vi "CreateProgram.vi"() -> ()   [LabVIEW 2018]
panel:
  out "error out":errorcluster
  in  "Clear":bool
  in  "Save":bool
  in  "Loop End":bool
  in  "Loop Start":bool
  in  "Incubate":bool
  in  "Change Reagent":bool
  in  "Feed":bool
  in  "Pump":bool
  out "Program Steps":i32(listbox)
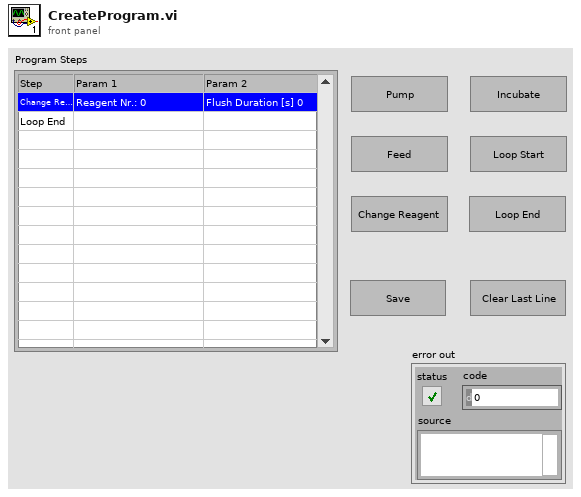
[diagram p1: front panel]
types:
  T1 = enum16{"open", "replace", "create", "open or create", "replace or create", "replace or create with confirmation"}
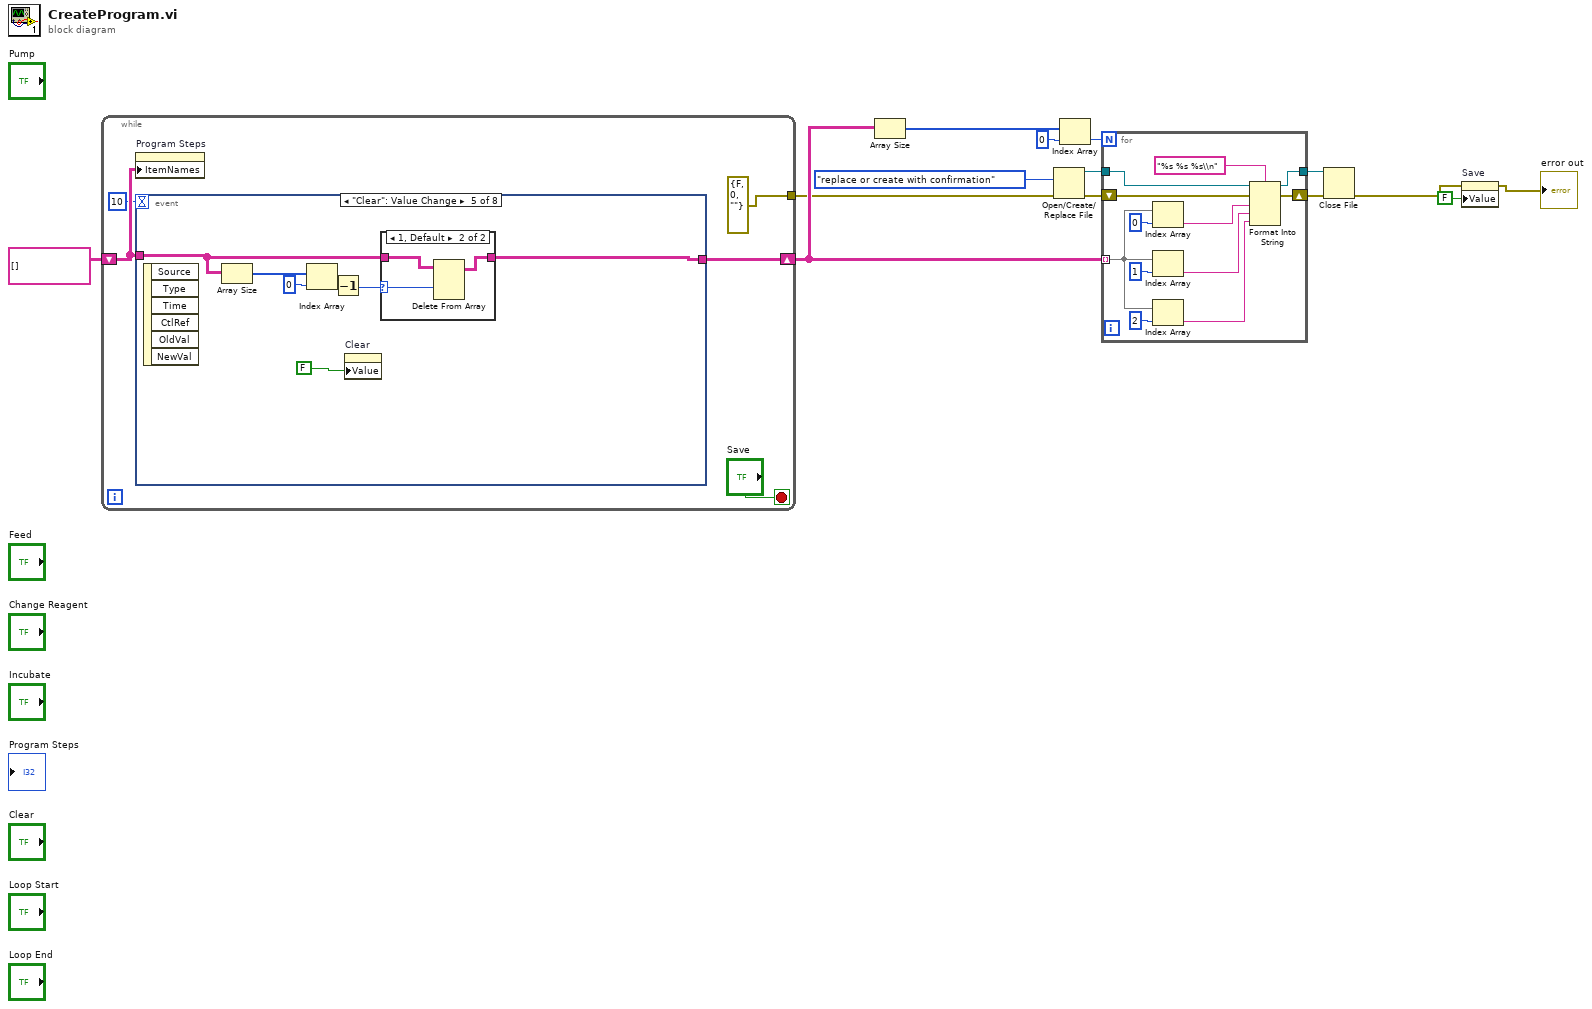
[diagram p0: block diagram]
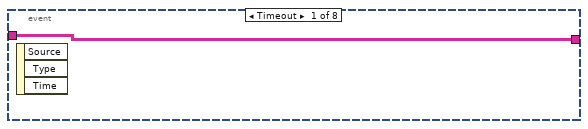
[diagram p2: hidden frame]
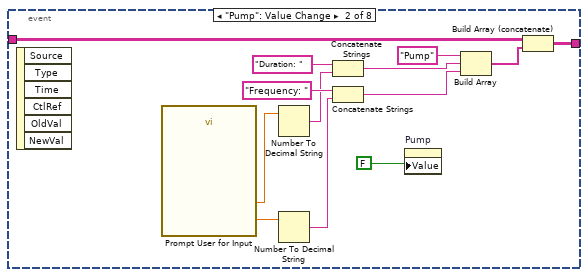
[diagram p3: hidden frame]
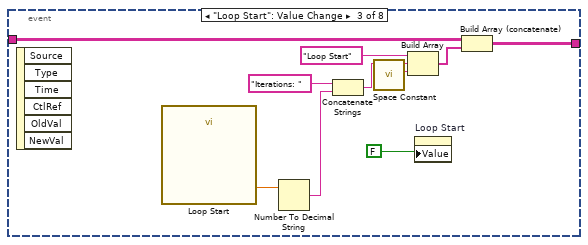
[diagram p4: hidden frame]
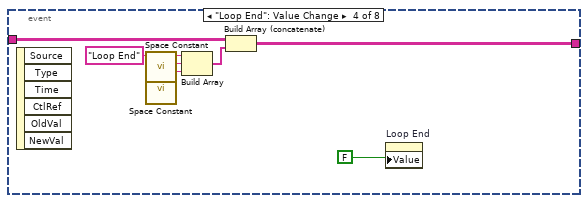
[diagram p5: hidden frame]
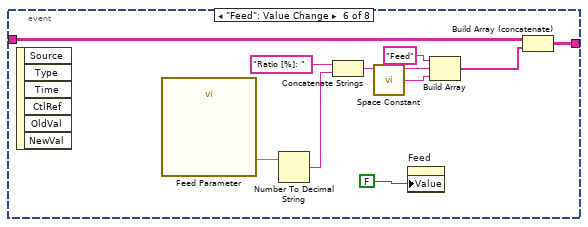
[diagram p7: hidden frame]
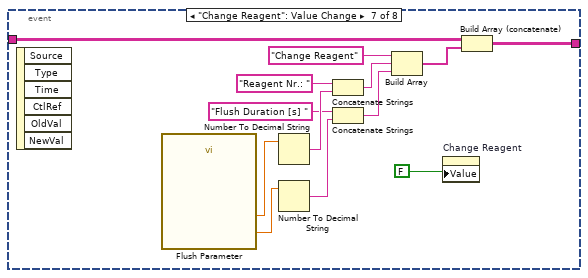
[diagram p8: hidden frame]
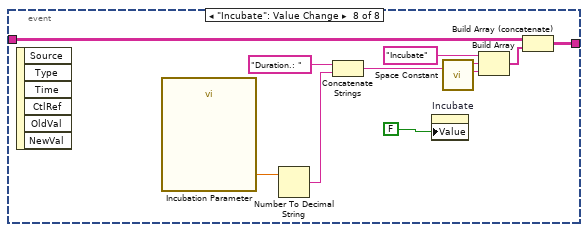
[diagram p9: hidden frame]
diagram:
  n1 = while {
    shift-right: [w17] -> w8
    shift-left: string[][] [] -> [w18]
    tunnel: [errorcluster {"status"=FALSE, "code"=0, "source"=""} ("error constant")] -> w4
    stop <- "Save" stop-if-true
    n2 = property on="Program Steps" class="MCListbox (strict)"("ItemNames"=w18) -> ()  [unwired: 2 in, 2 out]
    n3 = event shown="[4] \"Clear\": Value Change" {
      selector: _ -> [_ _ _ _ _ _ _ _]
      dyn-events: _ -> [_ _ _ _ _ _ _ _]
      timeout: 10 -> [_ _ _ _ _ _ _ _]
      tunnel: w18 -> [w20 w24 w36 w47 w56 w65 w78 w88]
      tunnel: [w20 w25 w37 w48 w57 w66 w79 w89] -> w17
      event Timeout {
        n4 = event-data() -> ()  [unwired: 1 in, 3 out]
      }
      event "Pump": Value Change {
        n5 = event-data() -> ()  [unwired: 1 in, 6 out]
        n6 = call "Prompt User for Input"() -> ("Frequency [Hz]"=w28:dbl, "Duration [s]"=w31:dbl)  [unwired: 16 in, 2 out]
        n7 = Number To Decimal String(number=w31) -> (decimal integer string=w22:string)  [unwired: 1 in]
        n8 = Number To Decimal String(number=w28) -> (decimal integer string=w23:string)  [unwired: 1 in]
        n9 = Concatenate Strings("Duration: ", w22) -> (w30:string)
        n10 = Concatenate Strings("Frequency: ", w23) -> (w27:string)
        n11 = property on="Pump" class="Bool (strict)"("Value"=FALSE ("Value (Signaling)")) -> ()  [unwired: 2 in, 2 out]
        n12 = Build Array("Pump", w30, w27) -> (w26:string[])
        n13 = Build Array (concatenate)(w24, w26) -> (w25:string[][])
      }
      event "Loop Start": Value Change {
        n14 = event-data() -> ()  [unwired: 1 in, 6 out]
        n15 = call "Loop Start"() -> ("Iterations"=w41:dbl)  [unwired: 17 in, 2 out]
        n16 = Number To Decimal String(number=w41) -> (decimal integer string=w35:string)  [unwired: 1 in]
        n17 = Concatenate Strings("Iterations: ", w35) -> (w40:string)
        n18 = call <vilib>:"Space Constant.vi"() -> ("String"=w39:string)
        n19 = Build Array("Loop Start", w40, w39) -> (w38:string[])
        n20 = property on="Loop Start" class="Bool (strict)"("Value"=FALSE ("Value (Signaling)")) -> ()  [unwired: 2 in, 2 out]
        n21 = Build Array (concatenate)(w36, w38) -> (w37:string[][])
      }
      event "Loop End": Value Change {
        n22 = event-data() -> ()  [unwired: 1 in, 6 out]
        n23 = call <vilib>:"Space Constant.vi"() -> ("String"=w46:string)
        n24 = call <vilib>:"Space Constant.vi"() -> ("String"=w45:string)
        n25 = Build Array("Loop End", w46, w45) -> (w49:string[])
        n26 = Build Array (concatenate)(w47, w49) -> (w48:string[][])
        n27 = property on="Loop End" class="Bool (strict)"("Value"=FALSE ("Value (Signaling)")) -> ()  [unwired: 2 in, 2 out]
      }
      event "Clear": Value Change {
        n28 = event-data() -> ()  [unwired: 1 in, 6 out]
        n29 = Array Size(array=w56) -> (size(s)=w55:i32[])
        n30 = Index Array(array=w55, index=0) -> (element=w53:i32)
        n31 = Decrement(x=w53) -> (x-1=w52:i32)
        n32 = property on="Clear" class="Bool (strict)"("Value"=FALSE ("Value (Signaling)")) -> ()  [unwired: 2 in, 2 out]
        n33 = case shown="1, Default" w52 {
          selector: w52 -> [_ w59]
          tunnel: [w58 w61] -> w57
          tunnel: w56 -> [w58 w60]
          frame -1 {
          }
          frame 1, Default {
            n34 = Delete From Array(array=w60, index (row)=w59) -> (array with subset deleted=w61:string[][])  [unwired: 2 in, 1 out]
          }
        }
      }
      event "Feed": Value Change {
        n35 = event-data() -> ()  [unwired: 1 in, 6 out]
        n36 = call "Feed Parameter"() -> ("Ratio [%]"=w69:dbl)  [unwired: 17 in, 2 out]
        n37 = Number To Decimal String(number=w69) -> (decimal integer string=w64:string)  [unwired: 1 in]
        n38 = Concatenate Strings("Ratio [%]: ", w64) -> (w68:string)
        n39 = call <vilib>:"Space Constant.vi"() -> ("String"=w63:string)
        n40 = property on="Feed" class="Bool (strict)"("Value"=FALSE ("Value (Signaling)")) -> ()  [unwired: 2 in, 2 out]
        n41 = Build Array("Feed", w68, w63) -> (w67:string[])
        n42 = Build Array (concatenate)(w65, w67) -> (w66:string[][])
      }
      event "Change Reagent": Value Change {
        n43 = event-data() -> ()  [unwired: 1 in, 6 out]
        n44 = call "Flush Parameter"() -> ("Flush Duration [s]"=w75:dbl, "Reagent Nr."=w82:dbl)  [unwired: 16 in, 2 out]
        n45 = Number To Decimal String(number=w82) -> (decimal integer string=w77:string)  [unwired: 1 in]
        n46 = Number To Decimal String(number=w75) -> (decimal integer string=w76:string)  [unwired: 1 in]
        n47 = Concatenate Strings("Reagent Nr.: ", w77) -> (w81:string)
        n48 = Concatenate Strings("Flush Duration [s] ", w76) -> (w73:string)
        n49 = Build Array("Change Reagent", w81, w73) -> (w80:string[])
        n50 = property on="Change Reagent" class="Bool (strict)"("Value"=FALSE ("Value (Signaling)")) -> ()  [unwired: 2 in, 2 out]
        n51 = Build Array (concatenate)(w78, w80) -> (w79:string[][])
      }
      event "Incubate": Value Change {
        n52 = event-data() -> ()  [unwired: 1 in, 6 out]
        n53 = call "Incubation Parameter"() -> ("Duration [s]"=w92:dbl)  [unwired: 17 in, 2 out]
        n54 = Number To Decimal String(number=w92) -> (decimal integer string=w87:string)  [unwired: 1 in]
        n55 = Concatenate Strings("Duration.: ", w87) -> (w91:string)
        n56 = property on="Incubate" class="Bool (strict)"("Value"=FALSE ("Value (Signaling)")) -> ()  [unwired: 2 in, 2 out]
        n57 = call <vilib>:"Space Constant.vi"() -> ("String"=w86:string)
        n58 = Build Array("Incubate", w91, w86) -> (w90:string[])
        n59 = Build Array (concatenate)(w88, w90) -> (w89:string[][])
      }
    }
  }
  n60 = Array Size(array=w8) -> (size(s)=w11:i32[])
  n61 = Open/Create/Replace File(error in=w4, operation (0:open)=T1."replace or create with confirmation") -> (refnum out=w12:refnum<file>, error out=w5:errorcluster)  [unwired: 4 in, 1 out]
  n62 = Index Array(array=w11, index=0) -> (element=w10:i32)
  n63 = for {
    N: w10 -> [_]
    tunnel: w12 -> [w106]
    tunnel: w8 -> [w98] mode=indexing
    tunnel: [w97] -> w7
    shift-right: [w96] -> w6
    shift-left: w5 -> [w95]
    n64 = Index Array(array=w98, index=0) -> (element=w101:string)
    n65 = Index Array(array=w98, index=1) -> (element=w100:string)
    n66 = Index Array(array=w98, index=2) -> (element=w99:string)
    n67 = Format Into String(format string="%s %s %s\\n", initial string=w106, error in=w95, w101, w100, w99) -> (resulting string=w97:refnum<file>, error out=w96:errorcluster)
  }
  n68 = Close File(refnum=w7, error in=w6) -> (error out=w2:errorcluster)  [unwired: 1 out]
  n69 = property on="Save" class="Bool (strict)"(error in=w2, "Value"=FALSE ("Save")) -> (error out=→"error out":errorcluster)  [unwired: 1 in, 1 out]
